vi "ManualTresholdControl.vi"() -> ()   [LabVIEW 2012]
uses:
  <vilib>/Utility/NIReport.llb/NI_report.lvclass
  <vilib>/Utility/NIReport.llb/HTML/NI_HTML.lvclass
panel:
  out "IPR_count":u32
  in  "Channel":i8=6
  in  "Instrument VISA in":T1={"AWG VISA"="AgilentGenerator1", "Oscilloscope  VISA "="AgilentOsciloscope", "Integration Board IP"="172.16.17.47", "connection ID"=refnum, "report out"=refnum, "report file path"=path "C:/Documents and Settings/CTA_LAB01/Desktop/L0_Asic/L0 Asic Test Data"}
  in  "Amp Scaler":dbl(slide)=1.716326530612245 scale=0.1..10.0
  in  "Voltage Input":dbl(slide)=0.21071428571428574 scale=0.05..0.8
  in  "Treshold":i16(slide)=557 min=0 max=1000 scale=0.0..1000.0
  in  "stop":bool
  out "error out":errorcluster
  in  "error in":errorcluster
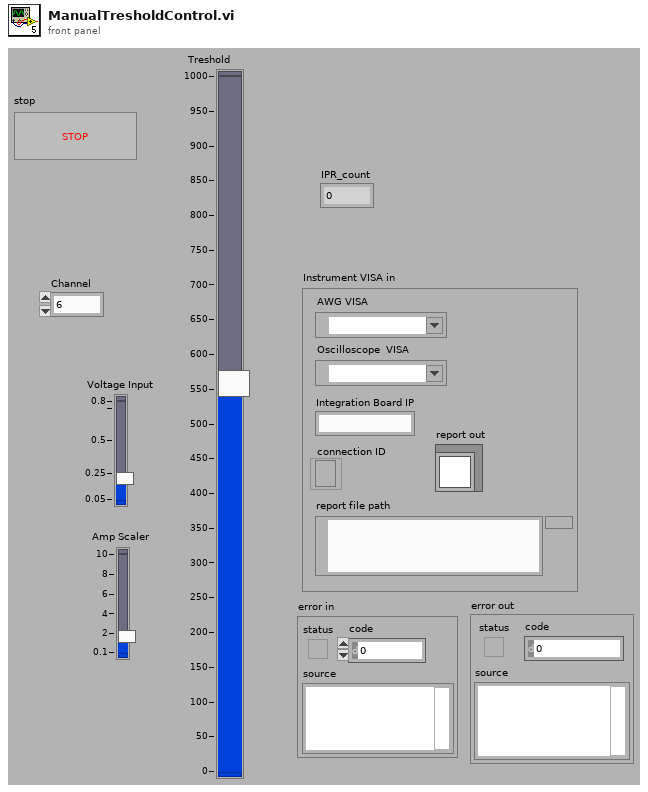
[diagram p1: front panel]
types:
  T1 = cluster{"AWG VISA":refnum<visa-resource-name>, "Oscilloscope  VISA ":refnum<visa-resource-name>, "Integration Board IP":string, "connection ID":refnum<k5>, "report out":refnum<class "NI_report.lvclass">, "report file path":path}
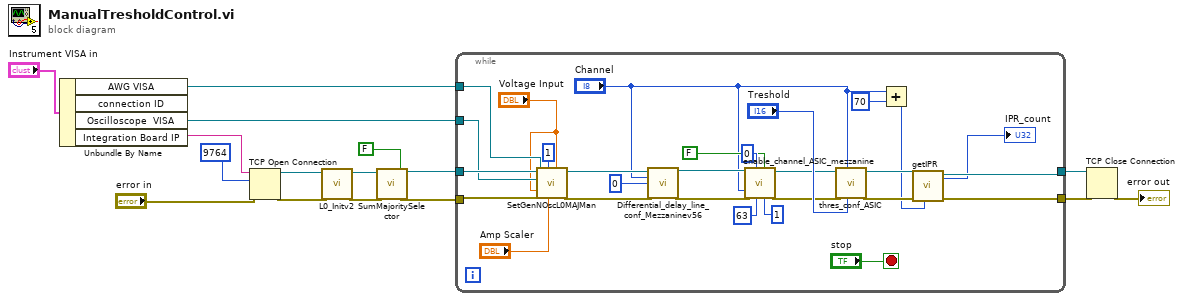
[diagram p0: block diagram]
diagram:
  n1 = Unbundle By Name("Instrument VISA in") -> ("AWG VISA"=w2:refnum<visa-resource-name>, "Oscilloscope  VISA"=w3:refnum<visa-resource-name>, "Integration Board IP"=w11:string)  [unwired: 1 out]
  n2 = TCP Open Connection(address=w11, remote port or service name=u16 9764, error in (no error)="error in") -> (connection ID=w10:refnum<k5>, error out=w9:errorcluster)  [unwired: 2 in]
  n3 = call "L0_Initv2.vi"("error in"=w9, "connection ID in"=w10) -> ("error out"=w8:errorcluster, "connection ID out"=w7:refnum<k5>)  [unwired: 8 in]
  n4 = call "SumMajoritySelector.vi"("On Sum\nOff Majority"=FALSE ("On Sum\nOff Majority"), "error in (no error)"=w8, "connection ID"=w7) -> ("error out"=w5:errorcluster, "connection ID out"=w6:refnum<k5>)  [unwired: 5 in]
  n5 = while {
    tunnel: [w23] -> w14
    tunnel: [w21] -> w13
    tunnel: w5 -> [w38]
    tunnel: w6 -> [w28]
    tunnel: w3 -> [w26]
    tunnel: w2 -> [w39]
    stop <- "stop" stop-if-true
    n6 = call "SetGenNOscL0MAJMan.vi"("Input Voltage"="Voltage Input", "Amp Scaler"="Amp Scaler", "NChannels"=1, "error in (no error)"=w38, "Output Voltage"="Voltage Input", "VISA resource name"=w26, "AWG VISA"=w39) -> ("error out 2"=w37:errorcluster)  [unwired: 4 in]
    n7 = call "Differential_delay_line_conf_Mezzaninev56.vi"("connection ID"=w28, "channel"="Channel", "Delay value"=u16 0, "error in (no error)"=w37) -> ("connection ID out"=w33:refnum<k5>, "error out 2"=w35:errorcluster)  [unwired: 4 in, 6 out]
    n8 = call "enable_channel_ASIC_mezzanine.vi"("Clip_sel_b"=u32 1, "maj/sum"=FALSE, "Ib_clipVb"=u32 63, "Att gain"=u32 0, "error in"=w35, "Channel"="Channel", "connection ID"=w33) -> ("error out"=w34:errorcluster, "connection ID out"=w32:refnum<k5>)  [unwired: 2 in, 1 out]
    n9 = call "thres_conf_ASIC.vi"("threshold"="Treshold", "Ring"="Channel", "error out 3"=w34, "connection ID"=w32) -> ("error out 2"=w25:errorcluster, "connection ID out"=w22:refnum<k5>)  [unwired: 4 in, 2 out]
    n10 = Add(x="Channel", y=i8 70) -> (x+y=w17:i8)
    n11 = call "getIPR.vi"("Address"=w17, "error in"=w25, "connection ID"=w22) -> ("error out"=w23:errorcluster, "connection ID out"=w21:refnum<k5>, "IPR_count"=→"IPR_count":u32)  [unwired: 5 in, 1 out]
  }
  n12 = TCP Close Connection(connection ID=w13, error in (no error)=w14) -> (error out=→"error out":errorcluster)  [unwired: 1 in, 1 out]
